vi "nanocal -- nuclear schottky fit V5.vi"() -> ()   [LabVIEW 2020] (continued)
"IDS0315_210901_RAW_cal__sam_"="IDS0315_210901_RAW_cal_CeCoIn5_4th_044(130)_C(f)_12T_0.300K_45deg_Tdep_raw_.dat", "IDS0316_210901_RAW_cal__ref_"="IDS0316_210901_RAW_cal_CeCoIn5_4th_045(131)_C(f)_12T_0.360K_45deg_Tdep_raw_.dat", "IDS0316_210901_RAW_cal__sam_"="IDS0316_210901_RAW_cal_CeCoIn5_4th_045(131)_C(f)_12T_0.360K_45deg_Tdep_raw_.dat", "IDS0317_210901_RAW_cal__ref_"="IDS0317_210901_RAW_cal_CeCoIn5_4th_046(132)_C(f)_12T_0.43K_45deg_Tdep_raw_.dat", "IDS0317_210901_RAW_cal__sam_"="IDS0317_210901_RAW_cal_CeCoIn5_4th_046(132)_C(f)_12T_0.43K_45deg_Tdep_raw_.dat", "IDS0318_210901_RAW_cal__ref_"="IDS0318_210901_RAW_cal_CeCoIn5_4th_047(133)_C(f)_12T_0.53K_45deg_Tdep_raw_.dat", "IDS0318_210901_RAW_cal__sam_"="IDS0318_210901_RAW_cal_CeCoIn5_4th_047(133)_C(f)_12T_0.53K_45deg_Tdep_raw_.dat", "IDS0319_210901_RAW_cal__ref_"="IDS0319_210901_RAW_cal_CeCoIn5_4th_048(134)_C(f)_12T_0.62K_45deg_Tdep_raw_.dat", "IDS0319_210901_RAW_cal__sam_"="IDS0319_210901_RAW_cal_CeCoIn5_4th_048(134)_C(f)_12T_0.62K_45deg_Tdep_raw_.dat", "IDS0320_210901_RAW_cal__ref_"="IDS0320_210901_RAW_cal_CeCoIn5_4th_049(135)_C(f)_12T_0.83K_45deg_Tdep_raw_.dat", "IDS0320_210901_RAW_cal__sam_"="IDS0320_210901_RAW_cal_CeCoIn5_4th_049(135)_C(f)_12T_0.83K_45deg_Tdep_raw_.dat", "IDS0321_210901_RAW_cal__ref_"="IDS0321_210901_RAW_cal_CeCoIn5_4th_050(136)_C(f)_12T_1.13K_45deg_Tdep_raw_.dat", "IDS0321_210901_RAW_cal__sam_"="IDS0321_210901_RAW_cal_CeCoIn5_4th_050(136)_C(f)_12T_1.13K_45deg_Tdep_raw_.dat", "IDS0322_210901_RAW_cal__ref_"="IDS0322_210901_RAW_cal_CeCoIn5_4th_051(137)_C(f)_12T_1.90K_45deg_Tdep_raw_.dat", "IDS0322_210901_RAW_cal__sam_"="IDS0322_210901_RAW_cal_CeCoIn5_4th_051(137)_C(f)_12T_1.90K_45deg_Tdep_raw_.dat", "IDS0323_210901_RAW_cal__ref_"="IDS0323_210901_RAW_cal_CeCoIn5_4th_052(138)_C(f)_12T_3.10K_45deg_Tdep_raw_.dat", "IDS0323_210901_RAW_cal__sam_"="IDS0323_210901_RAW_cal_CeCoIn5_4th_052(138)_C(f)_12T_3.10K_45deg_Tdep_raw_.dat", "IDS0324_210901_RAW_cal__ref_"="IDS0324_210901_RAW_cal_CeCoIn5_4th_053(139)_C(f)_12T_5.70K_45deg_Tdep_raw_.dat", "IDS0324_210901_RAW_cal__sam_"="IDS0324_210901_RAW_cal_CeCoIn5_4th_053(139)_C(f)_12T_5.70K_45deg_Tdep_raw_.dat", "IDS0330_210901_RAW_cal__ref_"="IDS0330_210901_RAW_cal_CeCoIn5_4th_059_C(f)_1T_0.197K_90deg_Bdep_raw_.dat", "IDS0330_210901_RAW_cal__sam_"="IDS0330_210901_RAW_cal_CeCoIn5_4th_059_C(f)_1T_0.197K_90deg_Bdep_raw_.dat", "IDS0331_210901_RAW_cal__ref_"="IDS0331_210901_RAW_cal_CeCoIn5_4th_060_C(f)_2T_0.197K_90deg_Bdep_raw_.dat", "IDS0331_210901_RAW_cal__sam_"="IDS0331_210901_RAW_cal_CeCoIn5_4th_060_C(f)_2T_0.197K_90deg_Bdep_raw_.dat", "IDS0335_210904_RAW_cal__ref_"="IDS0335_210904_RAW_cal_CeCoIn5_4th_064_C(f)_5.0T_0.197K_90deg_fsweep_Tdep_raw_.dat", "IDS0335_210904_RAW_cal__sam_"="IDS0335_210904_RAW_cal_CeCoIn5_4th_064_C(f)_5.0T_0.197K_90deg_fsweep_Tdep_raw_.dat", "IDS0336_210904_RAW_cal__ref_"="IDS0336_210904_RAW_cal_CeCoIn5_4th_065_C(f)_5.0T_0.122K_90deg_fsweep_Tdep_raw_.dat", "IDS0336_210904_RAW_cal__sam_"="IDS0336_210904_RAW_cal_CeCoIn5_4th_065_C(f)_5.0T_0.122K_90deg_fsweep_Tdep_raw_.dat", "IDS0337_210904_RAW_cal__ref_"="IDS0337_210904_RAW_cal_CeCoIn5_4th_066_C(f)_5.0T_0.157K_90deg_Tdep_raw_.dat", "IDS0337_210904_RAW_cal__sam_"="IDS0337_210904_RAW_cal_CeCoIn5_4th_066_C(f)_5.0T_0.157K_90deg_Tdep_raw_.dat", "IDS0338_210904_RAW_cal__ref_"="IDS0338_210904_RAW_cal_CeCoIn5_4th_067_C(f)_5.0T_0.170K_90deg_Tdep_raw_.dat", "IDS0338_210904_RAW_cal__sam_"="IDS0338_210904_RAW_cal_CeCoIn5_4th_067_C(f)_5.0T_0.170K_90deg_Tdep_raw_.dat", "IDS0339_210904_RAW_cal__ref_"="IDS0339_210904_RAW_cal_CeCoIn5_4th_068_C(f)_5.0T_0.255K_90deg_Tdep_raw_.dat", "IDS0339_210904_RAW_cal__sam_"="IDS0339_210904_RAW_cal_CeCoIn5_4th_068_C(f)_5.0T_0.255K_90deg_Tdep_raw_.dat", "IDS0340_210904_RAW_cal__ref_"="IDS0340_210904_RAW_cal_CeCoIn5_4th_069_C(f)_5.0T_0.308K_90deg_Tdep_raw_.dat", "IDS0340_210904_RAW_cal__sam_"="IDS0340_210904_RAW_cal_CeCoIn5_4th_069_C(f)_5.0T_0.308K_90deg_Tdep_raw_.dat", "IDS0341_210904_RAW_cal__ref_"="IDS0341_210904_RAW_cal_CeCoIn5_4th_070_C(f)_5.0T_0.360K_90deg_Tdep_raw_.dat", "IDS0341_210904_RAW_cal__sam_"="IDS0341_210904_RAW_cal_CeCoIn5_4th_070_C(f)_5.0T_0.360K_90deg_Tdep_raw_.dat", "IDS0342_210904_RAW_cal__ref_"="IDS0342_210904_RAW_cal_CeCoIn5_4th_071_C(f)_5.0T_0.438K_90deg_Tdep_raw_.dat", "IDS0342_210904_RAW_cal__sam_"="IDS0342_210904_RAW_cal_CeCoIn5_4th_071_C(f)_5.0T_0.438K_90deg_Tdep_raw_.dat", "IDS0343_210904_RAW_cal__ref_"="IDS0343_210904_RAW_cal_CeCoIn5_4th_072_C(f)_5.0T_0.53K_90deg_Tdep_raw_.dat", "IDS0343_210904_RAW_cal__sam_"="IDS0343_210904_RAW_cal_CeCoIn5_4th_072_C(f)_5.0T_0.53K_90deg_Tdep_raw_.dat", "IDS0344_210904_RAW_cal__ref_"="IDS0344_210904_RAW_cal_CeCoIn5_4th_073_C(f)_5.0T_0.62K_90deg_Tdep_raw_.dat", "IDS0344_210904_RAW_cal__sam_"="IDS0344_210904_RAW_cal_CeCoIn5_4th_073_C(f)_5.0T_0.62K_90deg_Tdep_raw_.dat", "IDS0346_210904_RAW_cal__ref_"="IDS0346_210904_RAW_cal_CeCoIn5_4th_075_C(f)_8.0T_0.122K_90deg_Tdep_raw_.dat", "IDS0346_210904_RAW_cal__sam_"="IDS0346_210904_RAW_cal_CeCoIn5_4th_075_C(f)_8.0T_0.122K_90deg_Tdep_raw_.dat", "IDS0347_210906_RAW_cal__ref_"="IDS0347_210906_RAW_cal_CeCoIn5_4th_076_C(f)_8.0T_0.157K_90deg_Tdep_raw_.dat", "IDS0347_210906_RAW_cal__sam_"="IDS0347_210906_RAW_cal_CeCoIn5_4th_076_C(f)_8.0T_0.157K_90deg_Tdep_raw_.dat", "IDS0348_210906_RAW_cal__ref_"="IDS0348_210906_RAW_cal_CeCoIn5_4th_077_C(f)_8.0T_0.178K_90deg_Tdep_raw_.dat", "IDS0348_210906_RAW_cal__sam_"="IDS0348_210906_RAW_cal_CeCoIn5_4th_077_C(f)_8.0T_0.178K_90deg_Tdep_raw_.dat", "IDS0349_210906_RAW_cal__ref_"="IDS0349_210906_RAW_cal_CeCoIn5_4th_078_C(f)_8.0T_0.20K_90deg_Tdep_raw_.dat", "IDS0349_210906_RAW_cal__sam_"="IDS0349_210906_RAW_cal_CeCoIn5_4th_078_C(f)_8.0T_0.20K_90deg_Tdep_raw_.dat", "IDS0350_210906_RAW_cal__ref_"="IDS0350_210906_RAW_cal_CeCoIn5_4th_079_C(f)_8.0T_0.26K_90deg_Tdep_raw_.dat", "IDS0350_210906_RAW_cal__sam_"="IDS0350_210906_RAW_cal_CeCoIn5_4th_079_C(f)_8.0T_0.26K_90deg_Tdep_raw_.dat", "IDS0351_210906_RAW_cal__ref_"="IDS0351_210906_RAW_cal_CeCoIn5_4th_080_C(f)_8.0T_0.31K_90deg_Tdep_raw_.dat", "IDS0351_210906_RAW_cal__sam_"="IDS0351_210906_RAW_cal_CeCoIn5_4th_080_C(f)_8.0T_0.31K_90deg_Tdep_raw_.dat", "IDS0352_210906_RAW_cal__ref_"="IDS0352_210906_RAW_cal_CeCoIn5_4th_081_C(f)_8.0T_0.36K_90deg_Tdep_raw_.dat", "IDS0352_210906_RAW_cal__sam_"="IDS0352_210906_RAW_cal_CeCoIn5_4th_081_C(f)_8.0T_0.36K_90deg_Tdep_raw_.dat", "IDS0353_210906_RAW_cal__ref_"="IDS0353_210906_RAW_cal_CeCoIn5_4th_082_C(f)_8.0T_0.438K_90deg_Tdep_raw_.dat", "IDS0353_210906_RAW_cal__sam_"="IDS0353_210906_RAW_cal_CeCoIn5_4th_082_C(f)_8.0T_0.438K_90deg_Tdep_raw_.dat", "IDS0354_210906_RAW_cal__ref_"="IDS0354_210906_RAW_cal_CeCoIn5_4th_083_C(f)_8.0T_0.53K_90deg_Tdep_raw_.dat", "IDS0354_210906_RAW_cal__sam_"="IDS0354_210906_RAW_cal_CeCoIn5_4th_083_C(f)_8.0T_0.53K_90deg_Tdep_raw_.dat", "IDS0355_210906_RAW_cal__ref_"="IDS0355_210906_RAW_cal_CeCoIn5_4th_085_C(f)_8.0T_0.83K_90deg_Tdep_raw_.dat", "IDS0355_210906_RAW_cal__sam_"="IDS0355_210906_RAW_cal_CeCoIn5_4th_085_C(f)_8.0T_0.83K_90deg_Tdep_raw_.dat", "IDS0359_210907_RAW_cal__ref_"="IDS0359_210907_RAW_cal_CeCoIn5_4th_089_C(f)_12.0T_0.12K_60deg_Tdep_raw_.dat", "IDS0359_210907_RAW_cal__sam_"="IDS0359_210907_RAW_cal_CeCoIn5_4th_089_C(f)_12.0T_0.12K_60deg_Tdep_raw_.dat", "IDS0360_210907_RAW_cal__ref_"="IDS0360_210907_RAW_cal_CeCoIn5_4th_090_C(f)_12.0T_0.15K_60deg_Tdep_raw_.dat", "IDS0360_210907_RAW_cal__sam_"="IDS0360_210907_RAW_cal_CeCoIn5_4th_090_C(f)_12.0T_0.15K_60deg_Tdep_raw_.dat", "IDS0361_210908_RAW_cal__ref_"="IDS0361_210908_RAW_cal_CeCoIn5_4th_091_C(f)_12.0T_0.168K_60deg_Tdep_raw_.dat", "IDS0361_210908_RAW_cal__sam_"="IDS0361_210908_RAW_cal_CeCoIn5_4th_091_C(f)_12.0T_0.168K_60deg_Tdep_raw_.dat", "IDS0362_210908_RAW_cal__ref_"="IDS0362_210908_RAW_cal_CeCoIn5_4th_092_C(f)_12.0T_0.197K_60deg_Tdep_raw_.dat", "IDS0362_210908_RAW_cal__sam_"="IDS0362_210908_RAW_cal_CeCoIn5_4th_092_C(f)_12.0T_0.197K_60deg_Tdep_raw_.dat", "IDS0363_210908_RAW_cal__ref_"="IDS0363_210908_RAW_cal_CeCoIn5_4th_093_C(f)_12.0T_0.25K_60deg_Tdep_raw_.dat", "IDS0363_210908_RAW_cal__sam_"="IDS0363_210908_RAW_cal_CeCoIn5_4th_093_C(f)_12.0T_0.25K_60deg_Tdep_raw_.dat", "IDS0364_210908_RAW_cal__ref_"="IDS0364_210908_RAW_cal_CeCoIn5_4th_094_C(f)_12.0T_0.307K_60deg_Tdep_raw_.dat", "IDS0364_210908_RAW_cal__sam_"="IDS0364_210908_RAW_cal_CeCoIn5_4th_094_C(f)_12.0T_0.307K_60deg_Tdep_raw_.dat", "IDS0365_210908_RAW_cal__ref_"="IDS0365_210908_RAW_cal_CeCoIn5_4th_095_C(f)_12.0T_0.36K_60deg_Tdep_raw_.dat", "IDS0365_210908_RAW_cal__sam_"="IDS0365_210908_RAW_cal_CeCoIn5_4th_095_C(f)_12.0T_0.36K_60deg_Tdep_raw_.dat", "IDS0366_210908_RAW_cal__ref_"="IDS0366_210908_RAW_cal_CeCoIn5_4th_096_C(f)_12.0T_0.43K_60deg_Tdep_raw_.dat", "IDS0366_210908_RAW_cal__sam_"="IDS0366_210908_RAW_cal_CeCoIn5_4th_096_C(f)_12.0T_0.43K_60deg_Tdep_raw_.dat", "IDS0367_210908_RAW_cal__ref_"="IDS0367_210908_RAW_cal_CeCoIn5_4th_097_C(f)_12.0T_0.53K_60deg_Tdep_raw_.dat", "IDS0367_210908_RAW_cal__sam_"="IDS0367_210908_RAW_cal_CeCoIn5_4th_097_C(f)_12.0T_0.53K_60deg_Tdep_raw_.dat", "IDS0368_210908_RAW_cal__ref_"="IDS0368_210908_RAW_cal_CeCoIn5_4th_098_C(f)_12.0T_0.63K_60deg_Tdep_raw_.dat", "IDS0368_210908_RAW_cal__sam_"="IDS0368_210908_RAW_cal_CeCoIn5_4th_098_C(f)_12.0T_0.63K_60deg_Tdep_raw_.dat", "IDS0369_210908_RAW_cal__ref_"="IDS0369_210908_RAW_cal_CeCoIn5_4th_099_C(f)_12.0T_0.83K_60deg_Tdep_raw_.dat", "IDS0369_210908_RAW_cal__sam_"="IDS0369_210908_RAW_cal_CeCoIn5_4th_099_C(f)_12.0T_0.83K_60deg_Tdep_raw_.dat", "IDS0370_210908_RAW_cal__ref_"="IDS0370_210908_RAW_cal_CeCoIn5_4th_100_C(f)_12.0T_1.13K_60deg_Tdep_raw_.dat", "IDS0370_210908_RAW_cal__sam_"="IDS0370_210908_RAW_cal_CeCoIn5_4th_100_C(f)_12.0T_1.13K_60deg_Tdep_raw_.dat", "IDS0371_210908_RAW_cal__ref_"="IDS0371_210908_RAW_cal_CeCoIn5_4th_101_C(f)_12.0T_1.90K_60deg_Tdep_raw_.dat", "IDS0371_210908_RAW_cal__sam_"="IDS0371_210908_RAW_cal_CeCoIn5_4th_101_C(f)_12.0T_1.90K_60deg_Tdep_raw_.dat", "IDS0372_210908_RAW_cal__ref_"="IDS0372_210908_RAW_cal_CeCoIn5_4th_102_C(f)_12.0T_3.11K_60deg_Tdep_raw_.dat", "IDS0372_210908_RAW_cal__sam_"="IDS0372_210908_RAW_cal_CeCoIn5_4th_102_C(f)_12.0T_3.11K_60deg_Tdep_raw_.dat", "IDS0373_210908_RAW_cal__ref_"="IDS0373_210908_RAW_cal_CeCoIn5_4th_103_C(f)_12.0T_5.75K_60deg_Tdep_raw_.dat", "IDS0373_210908_RAW_cal__sam_"="IDS0373_210908_RAW_cal_CeCoIn5_4th_103_C(f)_12.0T_5.75K_60deg_Tdep_raw_.dat", "IDS0377_210909_RAW_cal__ref_"="IDS0377_210909_RAW_cal_CeCoIn5_4th_107_C(f)_8.0T_0.197K_0deg_Tdep_raw_.dat", "IDS0377_210909_RAW_cal__sam_"="IDS0377_210909_RAW_cal_CeCoIn5_4th_107_C(f)_8.0T_0.197K_0deg_Tdep_raw_.dat", "IDS0378_210909_RAW_cal__ref_"="IDS0378_210909_RAW_cal_CeCoIn5_4th_108_C(f)_8.0T_0.122K_0deg_Tdep_raw_.dat", "IDS0378_210909_RAW_cal__sam_"="IDS0378_210909_RAW_cal_CeCoIn5_4th_108_C(f)_8.0T_0.122K_0deg_Tdep_raw_.dat", "IDS0379_210909_RAW_cal__ref_"="IDS0379_210909_RAW_cal_CeCoIn5_4th_109_C(f)_8.0T_0.148K_0deg_Tdep_raw_.dat", "IDS0379_210909_RAW_cal__sam_"="IDS0379_210909_RAW_cal_CeCoIn5_4th_109_C(f)_8.0T_0.148K_0deg_Tdep_raw_.dat", "IDS0380_210909_RAW_cal__ref_"="IDS0380_210909_RAW_cal_CeCoIn5_4th_110_C(f)_8.0T_0.168K_0deg_Tdep_raw_.dat", "IDS0380_210909_RAW_cal__sam_"="IDS0380_210909_RAW_cal_CeCoIn5_4th_110_C(f)_8.0T_0.168K_0deg_Tdep_raw_.dat", "IDS0381_210909_RAW_cal__ref_"="IDS0381_210909_RAW_cal_CeCoIn5_4th_111_C(f)_8.0T_0.25K_0deg_Tdep_raw_.dat", "IDS0381_210909_RAW_cal__sam_"="IDS0381_210909_RAW_cal_CeCoIn5_4th_111_C(f)_8.0T_0.25K_0deg_Tdep_raw_.dat", "IDS0382_210909_RAW_cal__ref_"="IDS0382_210909_RAW_cal_CeCoIn5_4th_112_C(f)_8.0T_0.30K_0deg_Tdep_raw_.dat", "IDS0382_210909_RAW_cal__sam_"="IDS0382_210909_RAW_cal_CeCoIn5_4th_112_C(f)_8.0T_0.30K_0deg_Tdep_raw_.dat", "IDS0383_210910_RAW_cal__ref_"="IDS0383_210910_RAW_cal_CeCoIn5_4th_113_C(f)_8.0T_0.36K_0deg_Tdep_raw_.dat", "IDS0383_210910_RAW_cal__sam_"="IDS0383_210910_RAW_cal_CeCoIn5_4th_113_C(f)_8.0T_0.36K_0deg_Tdep_raw_.dat", "IDS0384_210910_RAW_cal__ref_"="IDS0384_210910_RAW_cal_CeCoIn5_4th_114_C(f)_8.0T_0.43K_0deg_Tdep_raw_.dat", "IDS0384_210910_RAW_cal__sam_"="IDS0384_210910_RAW_cal_CeCoIn5_4th_114_C(f)_8.0T_0.43K_0deg_Tdep_raw_.dat", "IDS0385_210910_RAW_cal__ref_"="IDS0385_210910_RAW_cal_CeCoIn5_4th_115_C(f)_8.0T_0.53K_0deg_Tdep_raw_.dat", "IDS0385_210910_RAW_cal__sam_"="IDS0385_210910_RAW_cal_CeCoIn5_4th_115_C(f)_8.0T_0.53K_0deg_Tdep_raw_.dat", "IDS0386_210910_RAW_cal__ref_"="IDS0386_210910_RAW_cal_CeCoIn5_4th_116_C(f)_8.0T_0.63K_0deg_Tdep_raw_.dat", "IDS0386_210910_RAW_cal__sam_"="IDS0386_210910_RAW_cal_CeCoIn5_4th_116_C(f)_8.0T_0.63K_0deg_Tdep_raw_.dat", "IDS0387_210910_RAW_cal__ref_"="IDS0387_210910_RAW_cal_CeCoIn5_4th_117_C(f)_8.0T_0.83K_0deg_Tdep_raw_.dat", "IDS0387_210910_RAW_cal__sam_"="IDS0387_210910_RAW_cal_CeCoIn5_4th_117_C(f)_8.0T_0.83K_0deg_Tdep_raw_.dat", "IDS0388_210910_RAW_cal__ref_"="IDS0388_210910_RAW_cal_CeCoIn5_4th_118_C(f)_8.0T_1.13K_0deg_Tdep_raw_.dat", "IDS0388_210910_RAW_cal__sam_"="IDS0388_210910_RAW_cal_CeCoIn5_4th_118_C(f)_8.0T_1.13K_0deg_Tdep_raw_.dat", "IDS0389_210910_RAW_cal__ref_"="IDS0389_210910_RAW_cal_CeCoIn5_4th_119_C(f)_8.0T_1.52K_0deg_Tdep_raw_.dat", "IDS0389_210910_RAW_cal__sam_"="IDS0389_210910_RAW_cal_CeCoIn5_4th_119_C(f)_8.0T_1.52K_0deg_Tdep_raw_.dat", "IDS0390_210910_RAW_cal__ref_"="IDS0390_210910_RAW_cal_CeCoIn5_4th_120_C(f)_8.0T_1.90K_0deg_Tdep_raw_.dat", "IDS0390_210910_RAW_cal__sam_"="IDS0390_210910_RAW_cal_CeCoIn5_4th_120_C(f)_8.0T_1.90K_0deg_Tdep_raw_.dat", "IDS0391_210910_RAW_cal__ref_"="IDS0391_210910_RAW_cal_CeCoIn5_4th_121_C(f)_8.0T_1.25K_0deg_Tdep_raw_.dat", "IDS0391_210910_RAW_cal__sam_"="IDS0391_210910_RAW_cal_CeCoIn5_4th_121_C(f)_8.0T_1.25K_0deg_Tdep_raw_.dat", "IDS0392_210910_RAW_cal__ref_"="IDS0392_210910_RAW_cal_CeCoIn5_4th_122_C(f)_8.0T_1.39K_0deg_Tdep_raw_.dat", "IDS0392_210910_RAW_cal__sam_"="IDS0392_210910_RAW_cal_CeCoIn5_4th_122_C(f)_8.0T_1.39K_0deg_Tdep_raw_.dat", "IDS0393_210910_RAW_cal__ref_"="IDS0393_210910_RAW_cal_CeCoIn5_4th_123_C(f)_8.0T_3.11K_0deg_Tdep_raw_.dat", "IDS0393_210910_RAW_cal__sam_"="IDS0393_210910_RAW_cal_CeCoIn5_4th_123_C(f)_8.0T_3.11K_0deg_Tdep_raw_.dat", "IDS0394_210910_RAW_cal__ref_"="IDS0394_210910_RAW_cal_CeCoIn5_4th_124_C(f)_8.0T_5.75K_0deg_Tdep_raw_.dat", "IDS0394_210910_RAW_cal__sam_"="IDS0394_210910_RAW_cal_CeCoIn5_4th_124_C(f)_8.0T_5.75K_0deg_Tdep_raw_.dat", "IDS0395_210910_RAW_cal__ref_"="IDS0395_210910_RAW_cal_CeCoIn5_4th_125_C(f)_8.0T_1.31K_0deg_Tdep_raw_.dat", "IDS0395_210910_RAW_cal__sam_"="IDS0395_210910_RAW_cal_CeCoIn5_4th_125_C(f)_8.0T_1.31K_0deg_Tdep_raw_.dat"}
  out "temps&degs":map{string, map{T1, dbl}}(c390)
  out "mathematica thing":map{string, map{T1, dbl}}(c390)
  out "constrained filename lookup":map{i32, string}(c390)={0="IDS0346_210904_RAW_cal__ref_", 1="IDS0347_210906_RAW_cal__ref_", 2="IDS0348_210906_RAW_cal__ref_", 3="IDS0349_210906_RAW_cal__ref_", 4="IDS0350_210906_RAW_cal__ref_", 5="IDS0351_210906_RAW_cal__ref_", 6="IDS0352_210906_RAW_cal__ref_", 7="IDS0353_210906_RAW_cal__ref_", 8="IDS0354_210906_RAW_cal__ref_", 9="IDS0355_210906_RAW_cal__ref_"}
  out "filesnames lookup":map{i32, string}(c390)={0="IDS0183_210310_RAW_cal__sam_", 1="IDS0311_210901_RAW_cal__sam_", 2="IDS0359_210907_RAW_cal__sam_", 3="IDS0336_210904_RAW_cal__sam_", 4="IDS0346_210904_RAW_cal__sam_", 5="IDS0378_210909_RAW_cal__sam_", 6="IDS0158_210310_RAW_cal__sam_", 7="IDS0300_210427_RAW_cal__sam_", 8="IDS0184_210310_RAW_cal__sam_", 9="IDS0210_210310_RAW_cal__sam_", 10="IDS0379_210909_RAW_cal__sam_", 11="IDS0360_210907_RAW_cal__sam_", 12="IDS0310_210901_RAW_cal__sam_", 13="IDS0337_210904_RAW_cal__sam_", 14="IDS0347_210906_RAW_cal__sam_", 15="IDS0305_210831_RAW_cal__sam_", 16="IDS0361_210908_RAW_cal__sam_", 17="IDS0380_210909_RAW_cal__sam_", 18="IDS0159_210310_RAW_cal__sam_", 19="IDS0304_210831_RAW_cal__sam_", 20="IDS0312_210901_RAW_cal__sam_", 21="IDS0338_210904_RAW_cal__sam_", 22="IDS0348_210906_RAW_cal__sam_", 23="IDS0181_210310_RAW_cal__sam_", 24="IDS0185_210310_RAW_cal__sam_", 25="IDS0208_210310_RAW_cal__sam_", 26="IDS0209_210310_RAW_cal__sam_", 27="IDS0211_210310_RAW_cal__sam_", 28="IDS0212_210310_RAW_cal__sam_", 29="IDS0213_210310_RAW_cal__sam_", 30="IDS0214_210310_RAW_cal__sam_", 31="IDS0215_210310_RAW_cal__sam_", 32="IDS0216_210310_RAW_cal__sam_", 33="IDS0217_210310_RAW_cal__sam_", 34="IDS0330_210901_RAW_cal__sam_", 35="IDS0331_210901_RAW_cal__sam_", 36="IDS0335_210904_RAW_cal__sam_", 37="IDS0362_210908_RAW_cal__sam_", 38="IDS0377_210909_RAW_cal__sam_", 39="IDS0160_210310_RAW_cal__sam_", 40="IDS0303_210831_RAW_cal__sam_", 41="IDS0313_210901_RAW_cal__sam_", 42="IDS0349_210906_RAW_cal__sam_", 43="IDS0161_210310_RAW_cal__sam_", 44="IDS0186_210310_RAW_cal__sam_", 45="IDS0302_210831_RAW_cal__sam_", 46="IDS0363_210908_RAW_cal__sam_", 47="IDS0381_210909_RAW_cal__sam_", 48="IDS0314_210901_RAW_cal__sam_", 49="IDS0339_210904_RAW_cal__sam_", 50="IDS0350_210906_RAW_cal__sam_", 51="IDS0162_210310_RAW_cal__sam_", 52="IDS0187_210310_RAW_cal__sam_", 53="IDS0301_210831_RAW_cal__sam_", 54="IDS0315_210901_RAW_cal__sam_", 55="IDS0382_210909_RAW_cal__sam_", 56="IDS0364_210908_RAW_cal__sam_", 57="IDS0340_210904_RAW_cal__sam_", 58="IDS0351_210906_RAW_cal__sam_", 59="IDS0163_210310_RAW_cal__sam_", 60="IDS0188_210310_RAW_cal__sam_", 61="IDS0299_210427_RAW_cal__sam_", 62="IDS0316_210901_RAW_cal__sam_", 63="IDS0341_210904_RAW_cal__sam_", 64="IDS0352_210906_RAW_cal__sam_", 65="IDS0365_210908_RAW_cal__sam_", 66="IDS0383_210910_RAW_cal__sam_", 67="IDS0164_210310_RAW_cal__sam_", 68="IDS0189_210310_RAW_cal__sam_", 69="IDS0298_210427_RAW_cal__sam_", 70="IDS0317_210901_RAW_cal__sam_", 71="IDS0366_210908_RAW_cal__sam_", 72="IDS0384_210910_RAW_cal__sam_", 73="IDS0342_210904_RAW_cal__sam_", 74="IDS0353_210906_RAW_cal__sam_", 75="IDS0165_210310_RAW_cal__sam_", 76="IDS0190_210310_RAW_cal__sam_", 77="IDS0297_210427_RAW_cal__sam_", 78="IDS0318_210901_RAW_cal__sam_", 79="IDS0343_210904_RAW_cal__sam_", 80="IDS0354_210906_RAW_cal__sam_", 81="IDS0367_210908_RAW_cal__sam_", 82="IDS0385_210910_RAW_cal__sam_", 83="IDS0166_210310_RAW_cal__sam_", 84="IDS0191_210310_RAW_cal__sam_", 85="IDS0296_210427_RAW_cal__sam_", 86="IDS0319_210901_RAW_cal__sam_", 87="IDS0344_210904_RAW_cal__sam_", 88="IDS0368_210908_RAW_cal__sam_", 89="IDS0386_210910_RAW_cal__sam_", 90="IDS0220_210310_RAW_cal__sam_", 91="IDS0167_210310_RAW_cal__sam_", 92="IDS0192_210310_RAW_cal__sam_", 93="IDS0295_210427_RAW_cal__sam_", 94="IDS0320_210901_RAW_cal__sam_", 95="IDS0355_210906_RAW_cal__sam_", 96="IDS0369_210908_RAW_cal__sam_", 97="IDS0387_210910_RAW_cal__sam_", 98="IDS0168_210310_RAW_cal__sam_", 99="IDS0219_210310_RAW_cal__sam_", 100="IDS0193_210310_RAW_cal__sam_", 101="IDS0294_210427_RAW_cal__sam_", 102="IDS0321_210901_RAW_cal__sam_", 103="IDS0370_210908_RAW_cal__sam_", 104="IDS0388_210910_RAW_cal__sam_", 105="IDS0169_210310_RAW_cal__sam_", 106="IDS0391_210910_RAW_cal__sam_", 107="IDS0395_210910_RAW_cal__sam_", 108="IDS0392_210910_RAW_cal__sam_", 109="IDS0389_210910_RAW_cal__sam_", 110="IDS0218_210310_RAW_cal__sam_", 111="IDS0194_210310_RAW_cal__sam_", 112="IDS0293_210427_RAW_cal__sam_", 113="IDS0322_210901_RAW_cal__sam_", 114="IDS0371_210908_RAW_cal__sam_", 115="IDS0390_210910_RAW_cal__sam_", 116="IDS0170_210310_RAW_cal__sam_", 117="IDS0195_210310_RAW_cal__sam_", 118="IDS0306_210831_RAW_cal__sam_", 119="IDS0323_210901_RAW_cal__sam_", 120="IDS0372_210908_RAW_cal__sam_", 121="IDS0393_210910_RAW_cal__sam_", 122="IDS0171_210310_RAW_cal__sam_", 123="IDS0196_210310_RAW_cal__sam_", 124="IDS0324_210901_RAW_cal__sam_", 125="IDS0373_210908_RAW_cal__sam_", 126="IDS0394_210910_RAW_cal__sam_", 127="IDS0172_210310_RAW_cal__sam_"}
  out "all full filenames":map{string, path}(c390)
  out "Plot:  goodness oscillations":cluster{"Array":i32[], "Array":dbl[]}(graph)={"Array"=[0, 1, 2, 3, 4, 5, 6, 7, 8, 9, 10, 11, 12, 13, 14, 15, 16, 17, 18, 19, 20, 21, 22, 23, 24, 25, 26, 27, 28, 29, 30, 31, 32, 33, 34, 35, 36, 37, 38, 39, 40, 41, 42, 43, 44, 45, 46, 47, 48, 49, 50, 51, 52, 53, 54, 55, 56, 57, 58, 59, 60, 61, 62, 63, 64, 65, 66, 67, 68, 69, 70, 71, 72, 73, 74, 75, 76, 77, 78, 79, 80, 81, 82, 83, 84, 85, 86, 87, 88, 89, 90, 91, 92, 93, 94, 95, 96, 97, 98, 99], "Array"=[4.89160795202892e-13, 4.585507321075433e-13, 4.2862501742346737e-13, 3.993767122567604e-13, 3.708144902248023e-13, 3.4292620826326115e-13, 3.157253104790758e-13, 2.8920052116965245e-13, 2.633396972706592e-13, 2.38147609271655e-13, 2.136381349604477e-13, 1.897861208466356e-13, 1.665911332493497e-13, 1.440627131477079e-13, 1.221999931799722e-13, 1.009886618774658e-13, 8.043305604887863e-14, 6.053317569421068e-14, 4.127904615347511e-14, 2.2678473682313793e-14, 4.7232183442158515e-15, -1.2586286179949724e-14, -2.925567774147986e-14, -4.528712474471952e-14, -6.06736882957648e-14, -7.542490937373358e-14, -8.954816055339876e-14, -1.0304387551562932e-13, -1.1589947751522445e-13, -1.2813014538259893e-13, -1.3972937390471785e-13, -1.507210155293759e-13, -1.6108295253225435e-13, -1.7082038908378117e-13, -1.7994763665263314e-13, -1.8846512891967926e-13, -1.9634944711799385e-13, -2.0364092356839336e-13, -2.103174405465591e-13, -2.1638767166987094e-13, -2.218498822148529e-13, -2.2671361316062288e-13, -2.30968889847194e-13, -2.346256869345531e-13, -2.376939790826871e-13, -2.4015641905683616e-13, -2.420299204108911e-13, -2.4331925363441087e-13, -2.4401054093958763e-13, -2.441189611568362e-13, -2.436375753922526e-13, -2.425707204545269e-13, -2.4092706996103885e-13, -2.3870445550744357e-13, -2.358976729233131e-13, -2.3252840625209714e-13, -2.2856282838601416e-13, -2.240343327519767e-13, -2.1894291934998478e-13, -2.132799145626585e-13, -2.0704748679434282e-13, -2.0024650340677574e-13, -1.9289344427297905e-13, -1.8496619166863404e-13, -1.7649076644588035e-13, -1.6744765296561326e-13, -1.5785766790954447e-13, -1.4770996925594915e-13, -1.3701886847350409e-13, -1.2575921207180762e-13, -1.139583219456064e-13, -1.0161272864794846e-13, -8.872286585970279e-14, -7.52961061556423e-14, -6.131510230100723e-14, -4.6800670977509284e-14, -3.1748041695589535e-14, -1.6155913412641e-14, -3.122502256758253e-17, 1.6622120346809766e-14, 3.3814531036346906e-14, 5.152605772607011e-14, 6.976797611857322e-14, 8.853638308603529e-14, 1.0783127862845632e-13, 1.2764919329888436e-13, 1.4798795869297443e-13, 1.6884844217246453e-13, 1.9022327116258175e-13, 2.1210810885463616e-13, 2.345124962277456e-13, 2.574234228558403e-13, 2.8085476652672803e-13, 3.04791782090863e-13, 3.2923924003780414e-13, 3.541858646649576e-13, 3.7964206431317926e-13, 4.055926601520543e-13, 4.3204285635201067e-13, 4.590078317434632e-13]}
  in  "# osccilation steps":i32=100
  out "log(|dlogG/dlogα|)":dbl[](array[slide])=[2.460514015130688e-05, 0.00014759937241804586, 5.706163551111754e-05, 0.00018806874474486314, 2.3225143166879937e-06, 4.63149141549737e-06] scale=1e-06..10.0 scale format="%#_2p"
  out "side map from NUM":map{i32, T8}(c390)={4000=enum."ref", 8000=enum."sam"}
  out "side map to STR":map{T8, string}(c390)={enum."sam"="_sam_", enum."ref"="_ref_"}
  out "side map to NUM":map{T8, i32}(c390)={enum."sam"=8000, enum."ref"=4000}
  out "data file parameters map":map{T1, T9}(c390)={enum."T (K)"=enum."get T", enum."B (T)"=enum."get B", enum."θ (deg)"=enum."get deg", enum."set of (B|T)"=enum."get change"}
  in  "cursor index map":map{T1, i32}(c390)={enum."ζ"=0, enum."τ1"=1, enum."τS"=2, enum."τN"=3, enum."τC"=4, enum."κ0"=5, enum."m1"=6, enum."m2"=7, enum."m3"=8}
  out "new selector names":map{T1, map{T10, string}}(c390)={enum."ζ"={enum."name"="ζ", enum."nameL"="zeta", enum."units"="sec", enum."prec"="%_4p"}, enum."τ1"={enum."name"="τ1", enum."nameL"="tau1", enum."units"="sec", enum."prec"="%_4p"}, enum."τS"={enum."name"="τS", enum."nameL"="tauS", enum."units"="sec", enum."prec"="%_4p"}, enum."τN"={enum."name"="τN", enum."nameL"="tauN", enum."units"="sec", enum."prec"="%_4p"}, enum."τC"={enum."name"="τC", enum."nameL"="tauC", enum."units"="sec", enum."prec"="%_4p"}, enum."κ0"={enum."name"="κ0", enum."nameL"="kappa0", enum."units"="WperK", enum."prec"="%_5p"}, enum."T (K)"={enum."name"="T", enum."nameL"="T", enum."units"="K", enum."prec"="%_4p"}, enum."B (T)"={enum."name"="B", enum."nameL"="B", enum."units"="T", enum."prec"="%_2p"}, enum."θ (deg)"={enum."name"="θ", enum."nameL"="theta", enum."units"="deg", enum."prec"="%_2p"}, enum."side (S|R)"={enum."name"="side", enum."nameL"="side", enum."units"="side", enum."prec"="%d"}}
  out "state of all selectors string":string="__8.0T__90deg__4000side_"
  out "state of all selectors":map{T1, map{bool, dbl}}(c390)={enum."T (K)"={TRUE=0.179}, enum."B (T)"={FALSE=8.0}, enum."θ (deg)"={FALSE=90.0}, enum."side (S|R)"={FALSE=4000.0}, enum."set of (B|T)"={FALSE=1.0}}
  in  "tab 7":enum32{"Page 1"}(tab)
  in  "tab 3":enum32{"Page 1"}(tab)
  out "key":string="IDS0351_210906_RAW_cal__ref_"
  out "T (K)":dbl=0.31 format="%#_10f"
  out "θ (deg)":dbl=90.0 format="%#_10f"
  out "B (T)":dbl=8.0
  in  "tab 6":enum32{"Page 1"}(tab)
  in  "τ→Math! :p":bool
  in  "selection :|\\":u16(ring)=5 caption="files" items=["IDS0336_210904_RAW_cal_CeCoIn5_4th_065_C(f)_5.0T_0.122K_90deg_fsweep_Tdep_raw_.dat", "IDS0337_210904_RAW_cal_CeCoIn5_4th_066_C(f)_5.0T_0.157K_90deg_Tdep_raw_.dat", "IDS0338_210904_RAW_cal_CeCoIn5_4th_067_C(f)_5.0T_0.170K_90deg_Tdep_raw_.dat", "IDS0335_210904_RAW_cal_CeCoIn5_4th_064_C(f)_5.0T_0.197K_90deg_fsweep_Tdep_raw_.dat", "IDS0339_210904_RAW_cal_CeCoIn5_4th_068_C(f)_5.0T_0.255K_90deg_Tdep_raw_.dat", "IDS0340_210904_RAW_cal_CeCoIn5_4th_069_C(f)_5.0T_0.308K_90deg_Tdep_raw_.dat", "IDS0341_210904_RAW_cal_CeCoIn5_4th_070_C(f)_5.0T_0.360K_90deg_Tdep_raw_.dat", "IDS0342_210904_RAW_cal_CeCoIn5_4th_071_C(f)_5.0T_0.438K_90deg_Tdep_raw_.dat", "IDS0343_210904_RAW_cal_CeCoIn5_4th_072_C(f)_5.0T_0.53K_90deg_Tdep_raw_.dat", "IDS0344_210904_RAW_cal_CeCoIn5_4th_073_C(f)_5.0T_0.62K_90deg_Tdep_raw_.dat"]
  in  "tab 5":enum32{"Page 1"}(tab)
  in  "Math→τ! :q":bool
  in  "ω0 (rad/sec)":dbl(slide)=19.063235402868393 scale=0.001..50000.0 scale format="%#_2p"
  in  "offset Re\noffset Im":cluster{"Numeric":dbl, "Numeric":dbl}(slide)={"Numeric"=-7415841.584158415, "Numeric"=0.0} scale=-250000000.0..500000.0 scale format="%#_1p"
  in  "newton control 4":enum32{"default values "}(tab)
  in  "default selector":T11(array[cluster])=[{"Plost: sweep window"=enum."ζ", "used default"=FALSE}, {"Plost: sweep window"=enum."τ1", "used default"=FALSE}, {"Plost: sweep window"=enum."τS", "used default"=FALSE}, {"Plost: sweep window"=enum."τN", "used default"=FALSE}, {"Plost: sweep window"=enum."τC", "used default"=FALSE}, {"Plost: sweep window"=enum."κ0", "used default"=FALSE}]
  in  "default values string":string="\"0\"->   <|\"T\" -> 0.120000, \"τN\"-> 0.670097, \"τC\"-> 0.001215, \"ζ\"-> 0.368640, \"κ0\"-> 0.00000000044100|>   ,\n\"1\"->   <|\"T\" -> 0.220000, \"τN\"-> 0.057428, \"τC\"-> 0.001386, \"ζ\"-> 0.131633, \"κ0\"-> 0.00000000120283|>   ,\n\"2\"->   <|\"T\" -> 0.320000, \"τN\"-> 0.014576, \"τC\"-> 0.001971, \"ζ\"-> 0.063259, \"κ0\"-> 0.00000000186767|>   ,\n\"3\"->   <|\"T\" -> 0.420000, \"τN\"-> 0.005816, \"τC\"-> 0.002645, \"ζ\"-> 0.041943, \"κ0\"-> 0.00000000259214|>   ,\n\"4\"->   <|\"T\" -> 0.520000, \"τN\"-> 0.002807, \"τC\"-> 0.003188, \"ζ\"-> 0.030182, \"κ0\"-> 0.00000000339327|>   ,\n\"5\"->   <|\"T\" -> 0.620000, \"τN\"-> 0.001928, \"τC\"-> 0.003634, \"ζ\"-> 0.025126, \"κ0\"-> 0.00000000404950|>   ,\n\"6\"->   <|\"T\" -> 0.720000, \"τN\"-> 0.001251, \"τC\"-> 0.004021, \"ζ\"-> 0.023386, \"κ0\"-> 0.00000000484450|>   ,\n\"7\"->   <|\"T\" -> 0.820000, \"τN\"-> 0.000866, \"τC\"-> 0.004389, \"ζ\"-> 0.022054, \"κ0\"-> 0.00000000563624|>   ,\n\"8\"->   <|\"T\" -> 0.920000, \"τN\"-> 0.000673, \"τC\"-> 0.004723, \"ζ\"-> 0.021623, \"κ0\"-> 0.00000000639866|>   ,\n\"9\"->   <|\"T\" -> 1.020000, \"τN\"-> 0.000537, \"τC\"-> 0.005044, \"ζ\"-> 0.021243, \"κ0\"-> 0.00000000716107|>   ,\n\"10\"->   <|\"T\" -> 1.120000, \"τN\"-> 0.000431, \"τC\"-> 0.005344, \"ζ\"-> 0.020967, \"κ0\"-> 0.00000000793323|>   ,\n\"11\"->   <|\"T\" -> 1.220000, \"τN\"-> 0.000336, \"τC\"-> 0.005596, \"ζ\"-> 0.020955, \"κ0\"-> 0.00000000874437|>   ,\n\"12\"->   <|\"T\" -> 1.320000, \"τN\"-> 0.000267, \"τC\"-> 0.005838, \"ζ\"-> 0.020944, \"κ0\"-> 0.00000000955551|>   ,\n\"13\"->   <|\"T\" -> 1.420000, \"τN\"-> 0.000216, \"τC\"-> 0.006071, \"ζ\"-> 0.020934, \"κ0\"-> 0.00000001036666|>   ,\n\"14\"->   <|\"T\" -> 1.520000, \"τN\"-> 0.000177, \"τC\"-> 0.006297, \"ζ\"-> 0.020925, \"κ0\"-> 0.00000001117780|>   ,\n\"15\"->   <|\"T\" -> 1.620000, \"τN\"-> 0.000147, \"τC\"-> 0.006517, \"ζ\"-> 0.020916, \"κ0\"-> 0.00000001198894|>   ,\n\"16\"->   <|\"T\" -> 1.720000, \"τN\"-> 0.000123, \"τC\"-> 0.006730, \"ζ\"-> 0.020907, \"κ0\"-> 0.00000001280009|>   ,\n\"17\"->   <|\"T\" -> 1.820000, \"τN\"-> 0.000105, \"τC\"-> 0.006885, \"ζ\"-> 0.020876, \"κ0\"-> 0.00000001362415|>   ,\n\"18\"->   <|\"T\" -> 1.920000, \"τN\"-> 0.000091, \"τC\"-> 0.006831, \"ζ\"-> 0.020754, \"κ0\"-> 0.00000001449990|>   ,\n\"19\"->   <|\"T\" -> 2.020000, \"τN\"-> 0.000080, \"τC\"-> 0.006781, \"ζ\"-> 0.020639, \"κ0\"-> 0.00000001537565|>   ,\n\"20\"->   <|\"T\" -> 2.120000, \"τN\"-> 0.000070, \"τC\"-> 0.006733, \"ζ\"-> 0.020530, \"κ0\"-> 0.00000001625140|>   ,\n\"21\"->   <|\"T\" -> 2.220000, \"τN\"-> 0.000062, \"τC\"-> 0.006687, \"ζ\"-> 0.020427, \"κ0\"-> 0.00000001712715|>   ,\n\"22\"->   <|\"T\" -> 2.320000, \"τN\"-> 0.000056, \"τC\"-> 0.006644, \"ζ\"-> 0.020329, \"κ0\"-> 0.00000001800290|>   ,\n\"23\"->   <|\"T\" -> 2.420000, \"τN\"-> 0.000050, \"τC\"-> 0.006603, \"ζ\"-> 0.020235, \"κ0\"-> 0.00000001887865|>   ,\n\"24\"->   <|\"T\" -> 2.520000, \"τN\"-> 0.000045, \"τC\"-> 0.006564, \"ζ\"-> 0.020146, \"κ0\"-> 0.00000001975440|>   ,\n\"25\"->   <|\"T\" -> 2.620000, \"τN\"-> 0.000040, \"τC\"-> 0.006527, \"ζ\"-> 0.020060, \"κ0\"-> 0.00000002063015|>   ,\n\"26\"->   <|\"T\" -> 2.720000, \"τN\"-> 0.000037, \"τC\"-> 0.006491, \"ζ\"-> 0.019978, \"κ0\"-> 0.00000002150590|>   ,\n\"27\"->   <|\"T\" -> 2.820000, \"τN\"-> 0.000033, \"τC\"-> 0.006457, \"ζ\"-> 0.019899, \"κ0\"-> 0.00000002238165|>   ,\n\"28\"->   <|\"T\" -> 2.920000, \"τN\"-> 0.000030, \"τC\"-> 0.006424, \"ζ\"-> 0.019824, \"κ0\"-> 0.00000002325740|>   ,\n\"29\"->   <|\"T\" -> 3.020000, \"τN\"-> 0.000028, \"τC\"-> 0.006374, \"ζ\"-> 0.019852, \"κ0\"-> 0.00000002421662|>   ,\n\"30\"->   <|\"T\" -> 3.120000, \"τN\"-> 0.000026, \"τC\"-> 0.006255, \"ζ\"-> 0.020282, \"κ0\"-> 0.00000002550973|>   ,\n\"31\"->   <|\"T\" -> 3.220000, \"τN\"-> 0.000024, \"τC\"-> 0.006143, \"ζ\"-> 0.020708, \"κ0\"-> 0.00000002680284|>   ,\n\"32\"->   <|\"T\" -> 3.320000, \"τN\"-> 0.000023, \"τC\"-> 0.006036, \"ζ\"-> 0.021130, \"κ0\"-> 0.00000002809596|>   ,\n\"33\"->   <|\"T\" -> 3.420000, \"τN\"-> 0.000021, \"τC\"-> 0.005933, \"ζ\"-> 0.021547, \"κ0\"-> 0.00000002938907|>   ,\n\"34\"->   <|\"T\" -> 3.520000, \"τN\"-> 0.000020, \"τC\"-> 0.005836, \"ζ\"-> 0.021960, \"κ0\"-> 0.00000003068218|>   ,\n\"35\"->   <|\"T\" -> 3.620000, \"τN\"-> 0.000019, \"τC\"-> 0.005742, \"ζ\"-> 0.022368, \"κ0\"-> 0.00000003197529|>   ,\n\"36\"->   <|\"T\" -> 3.720000, \"τN\"-> 0.000018, \"τC\"-> 0.005653, \"ζ\"-> 0.022774, \"κ0\"-> 0.00000003326840|>   ,\n\"37\"->   <|\"T\" -> 3.820000, \"τN\"-> 0.000017, \"τC\"-> 0.005567, \"ζ\"-> 0.023175, \"κ0\"-> 0.00000003456151|>   ,\n\"38\"->   <|\"T\" -> 3.920000, \"τN\"-> 0.000016, \"τC\"-> 0.005485, \"ζ\"-> 0.023573, \"κ0\"-> 0.00000003585462|>   ,\n\"39\"->   <|\"T\" -> 4.020000, \"τN\"-> 0.000015, \"τC\"-> 0.005406, \"ζ\"-> 0.023967, \"κ0\"-> 0.00000003714773|>   ,\n\"40\"->   <|\"T\" -> 4.120000, \"τN\"-> 0.000014, \"τC\"-> 0.005330, \"ζ\"-> 0.024358, \"κ0\"-> 0.00000003844084|>   ,\n\"41\"->   <|\"T\" -> 4.220000, \"τN\"-> 0.000013, \"τC\"-> 0.005257, \"ζ\"-> 0.024746, \"κ0\"-> 0.00000003973396|>   ,\n\"42\"->   <|\"T\" -> 4.320000, \"τN\"-> 0.000013, \"τC\"-> 0.005186, \"ζ\"-> 0.025131, \"κ0\"-> 0.00000004102707|>   ,\n\"43\"->   <|\"T\" -> 4.420000, \"τN\"-> 0.000012, \"τC\"-> 0.005118, \"ζ\"-> 0.025512, \"κ0\"-> 0.00000004232018|>   ,\n\"44\"->   <|\"T\" -> 4.520000, \"τN\"-> 0.000012, \"τC\"-> 0.005053, \"ζ\"-> 0.025891, \"κ0\"-> 0.00000004361329|>   ,\n\"45\"->   <|\"T\" -> 4.620000, \"τN\"-> 0.000011, \"τC\"-> 0.004990, \"ζ\"-> 0.026267, \"κ0\"-> 0.00000004490640|>   ,\n\"46\"->   <|\"T\" -> 4.720000, \"τN\"-> 0.000011, \"τC\"-> 0.004928, \"ζ\"-> 0.026640, \"κ0\"-> 0.00000004619951|>   ,\n\"47\"->   <|\"T\" -> 4.820000, \"τN\"-> 0.000010, \"τC\"-> 0.004869, \"ζ\"-> 0.027010, \"κ0\"-> 0.00000004749262|>   ,\n\"48\"->   <|\"T\" -> 4.920000, \"τN\"-> 0.000010, \"τC\"-> 0.004812, \"ζ\"-> 0.027378, \"κ0\"-> 0.00000004878573|>   ,"
  in  "load default values":bool
  in  "selector":T12={"ignore set of !"=FALSE, "set (1T|2B)"=0, "ignore side !"=FALSE, "side (8S|4R)"=0, "ignore θ !"=FALSE, "ignore B !"=FALSE, "T (K)"=10, "ignore T !"=TRUE, "θ (deg)"=4, "B (T)"=6, "lookup"={"set of lookup"={0=1.0, 1=2.0}, "all set of"={1.0, 2.0}, "T lookup"={0=0.12, 1=0.122, 2=0.14, 3=0.148, 4=0.15, 5=0.157, 6=0.16, 7=0.168, 8=0.17, 9=0.178, 10=0.179, 11=0.197, 12=0.2, 13=0.22, 14=0.249, 15=0.25, 16=0.255, 17=0.26, 18=0.28, 19=0.3, 20=0.307, 21=0.308, 22=0.31, 23=0.33, 24=0.36, 25=0.4, 26=0.43, 27=0.438, 28=0.48, 29=0.512, 30=0.53, 31=0.58, 32=0.61, 33=0.62, 34=0.63, 35=0.677, 36=0.68, 37=0.81, 38=0.83, 39=0.91, 40=1.0, 41=1.1, 42=1.13, 43=1.23, 44=1.25, 45=1.31, 46=1.39, 47=1.52, 48=1.55, 49=1.8, 50=1.9, 51=1.97, 52=3.0, 53=3.1, 54=3.11, 55=3.19, 56=5.7, 57=5.75, 58=5.8}, "θ lookup"={0=0.0, 1=30.0, 2=45.0, 3=60.0, 4=90.0}, "B lookup"={0=0.0, 1=1.0, 2=2.0, 3=5.0, 4=6.0, 5=7.0, 6=8.0, 7=9.0, 8=10.0, 9=11.0, 10=12.0}, "all T's"={0.12, 0.122, 0.14, 0.148, 0.15, 0.157, 0.16, 0.168, 0.17, 0.178, 0.179, 0.197, 0.2, 0.22, 0.249, 0.25, 0.255, 0.26, 0.28, 0.3, 0.307, 0.308, 0.31, 0.33, 0.36, 0.4, 0.43, 0.438, 0.48, 0.512, 0.53, 0.58, 0.61, 0.62, 0.63, 0.677, 0.68, 0.81, 0.83, 0.91, 1.0, 1.1, 1.13, 1.23, 1.25, 1.31, 1.39, 1.52, 1.55, 1.8, 1.9, 1.97, 3.0, 3.1, 3.11, 3.19, 5.7, 5.75, 5.8}, "all θ's"={0.0, 30.0, 45.0, 60.0, 90.0}, "all B's"={0.0, 1.0, 2.0, 5.0, 6.0, 7.0, 8.0, 9.0, 10.0, 11.0, 12.0}, "all sides"={4000.0, 8000.0}, "side lookup"={0=4000.0, 1=8000.0}}} {"B (T)" items=["0.000", "1.000", "2.000", "5.000", "6.000", "7.000", "8.000", "9.000", "10.000", "11.000", "12.000"]; "θ (deg)" items=["0.000", "30.000", "45.000", "60.000", "90.000"]; "T (K)" items=["0.120", "0.122", "0.140", "0.148", "0.150", "0.157", "0.160", "0.168", "0.170", "0.178", "0.179", "0.197", "0.200", "0.220", "0.249", "0.250", "0.255", "0.260", "0.280", "0.300", "0.307", "0.308", "0.310", "0.330", "0.360", "0.400", "0.430", "0.438", "0.480", "0.512", "0.530", "0.580", "0.610", "0.620", "0.630", "0.677", "0.680", "0.810", "0.830", "0.910", "1.000", "1.100", "1.130", "1.230", "1.250", "1.310", "1.390", "1.520", "1.550", "1.800", "1.900", "1.970", "3.000", "3.100", "3.110", "3.190", "5.700", "5.750", "5.800"]; "side (8S|4R)" items=["4000", "8000"]; "set (1T|2B)" items=["1", "2"]}
  in  "parameter selectors 2":enum32{"Page 1"}(tab)
  in  "colors":u32[](array[colorbox])=[7087058, 56538, 2062078, 16740827, 16755712, 11121611, 8285330, 9272482, 9204890]
  in  "parameter":T1[](array[typedef])=[enum."ζ", enum."τ1", enum."τS", enum."τN", enum."τC", enum."κ0"]
  in  "overwrite offset":bool=TRUE
  in  "landscape plots":enum32{"Page 1", "Page 2"}(tab)
  in  "range one":dbl(slide)=0.006965 min=0.0 max=0.3 step=1e-06 scale=0.0001..1.0 scale format="%#_3p"
  in  "one":T1=enum."τS"
  out "Plot: goodness vs parameter":cluster{"Freq out (Hz)":dbl[], dbl[]}[](graph)
  in  "plot landscape!":bool
  in  "range two":dbl(slide)=0.0039049999999999996 min=0.0 max=0.3 step=1e-06 scale=0.0001..1.0 scale format="%#_3p"
  in  "two":T1=enum."τ1"
  in  "what":enum16{"1d plots", "2d plots "}(ring)
  in  "# points":i32=200
  in  "Array":T1[](array[typedef])=[enum."ζ", enum."τ1", enum."τS", enum."τN", enum."τC"]
  in  "color Map":map{T1, u32}(c390)={enum."ζ"=7087058, enum."τ1"=56538, enum."τS"=2062078, enum."τN"=16740827, enum."τC"=16755712, enum."κ0"=11121611}
